vi "Helmholtz2D_FEM_Check Input.vi"(0 "F(x, y)":dbl[](array[numeric]), 1 "Grid":cluster{"Xi":dbl[], "Yi":dbl[]}, 5 "k":dbl=1.0, 7 "a":dbl, 9 "Domain":cluster{"X":dbl[], "Y":dbl[]}, 11 "error in (no error)":errorcluster, 12 "Boundary Condition":cluster{"type":T1, "Value":dbl[]} {"type" items=["Dirichlet", "Neumann"]}) -> (15 "error out":errorcluster)   [LabVIEW 2017, in "NI_PDE.lvlib"]
uses:
  <vilib>/gmath/NI_PDE.lvlib
  <vilib>/gmath/pde.llb/Common/PDE_BC Type.ctl
  <vilib>/gmath/pde.llb/Common/PDE_Error.ctl
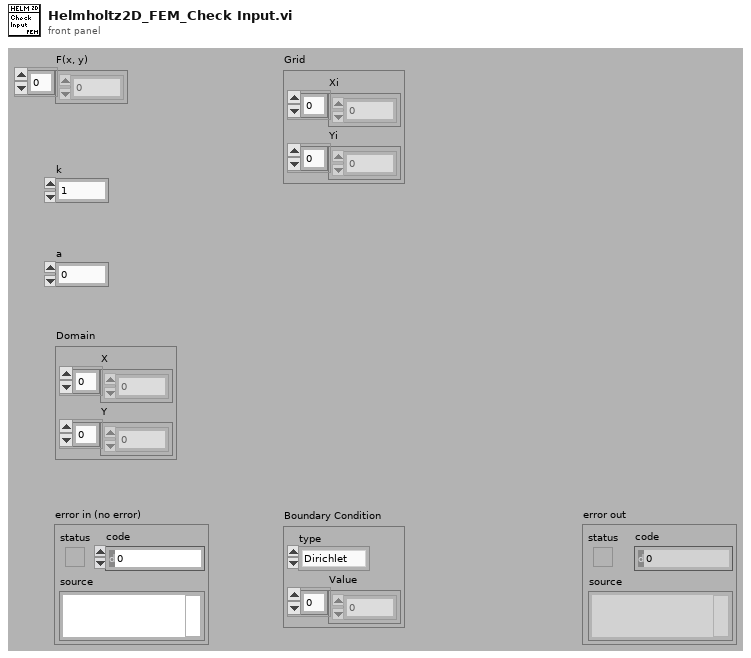
[diagram p1: front panel]
types:
  T1 = typedef "NI_PDE.lvlib/PDE_BC Type.ctl" = i32
  T2 = typedef "NI_PDE.lvlib/PDE_Error.ctl" = enum16{"No Error", "k is zero", "End point <= start point", "# of time steps < 2", "# of spatial points < 3", "# of grid < 1 for FEM", "# of boundary < 3 for FEM", "Incompatible RHS size", "Incompatible BC size", "Incompatible IC size", "PDE class conflict", "RHS class conflict", "Domain class conflict", "BC class conflict", "IC class conflict"}
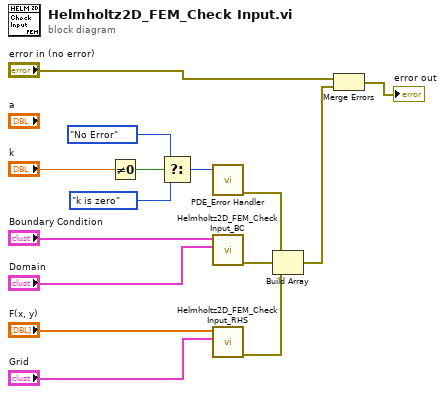
[diagram p0: block diagram]
diagram:
  n1 = Not Equal To 0?(x="k") -> (x != 0?=w15:bool)
  n2 = Select(t=PDE_Error."No Error" ("PDE error"), s=w15, f=PDE_Error."k is zero" ("PDE error")) -> (s? t:f=w12:T2)
  n3 = call <vilib>:"PDE_Error Handler.vi"("PDE error"=w12) -> ("error out"=w7:errorcluster)  [unwired: 1 in, 9 out]
  n4 = call <vilib>:"Helmholtz2D_FEM_Check Input_BC.vi"("Domain"="Domain", "Boundary Condition"="Boundary Condition") -> ("error out"=w2:errorcluster)  [unwired: 1 in, 8 out]
  n5 = call <vilib>:"Helmholtz2D_FEM_Check Input_RHS.vi"("Grid"="Grid", "F(x, y)"="F(x, y)") -> ("error out"=w1:errorcluster)  [unwired: 1 in, 8 out]
  n6 = Build Array(w7, w2, w1) -> (w10:errorcluster[])
  n7 = Merge Errors("error in (no error)", w10) -> (→"error out":errorcluster)
